vi "t값.vi"(5 "samples":i32=500, 7 "Time(S)":dbl=0.5, 8 "error in (no error)":errorcluster, 9 "c":dbl=0.001, 10 "r":dbl=40.0, 11 "v":dbl=800.0) -> (0 "error out":errorcluster, 2 "XY Graph":cluster{"Ramp Pattern":dbl[], dbl[]}[](graph), 3 "Waveform Graph":waveform(dbl)[](graph))   [LabVIEW 2019]
uses:
  <vilib>/Analysis/1siggen.llb/Ramp Pattern by Samples.vi
  <vilib>/Analysis/NI_AALBase.lvlib
panel:
  out "size(s) 2":i32
  out "size(s)":i32
  out "x/y":dbl
  out "output waveform":waveform(dbl)
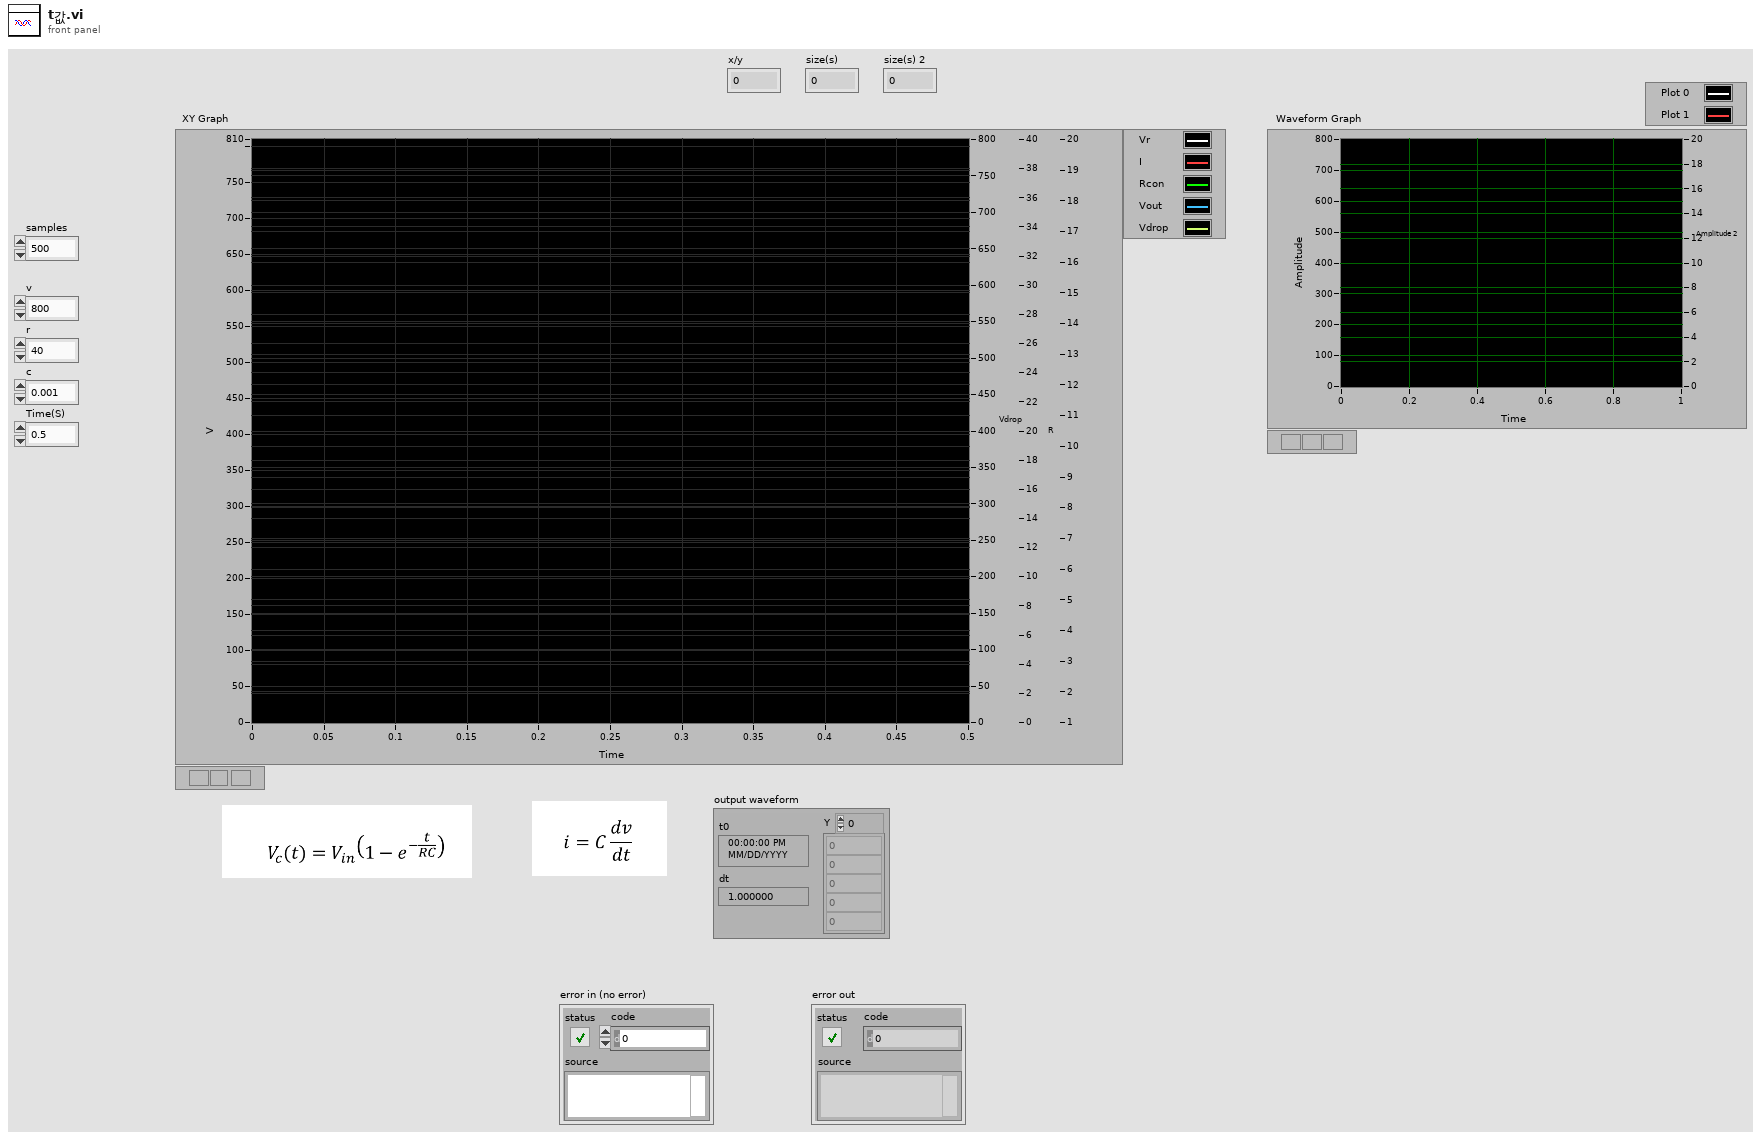
[diagram p1: front panel]
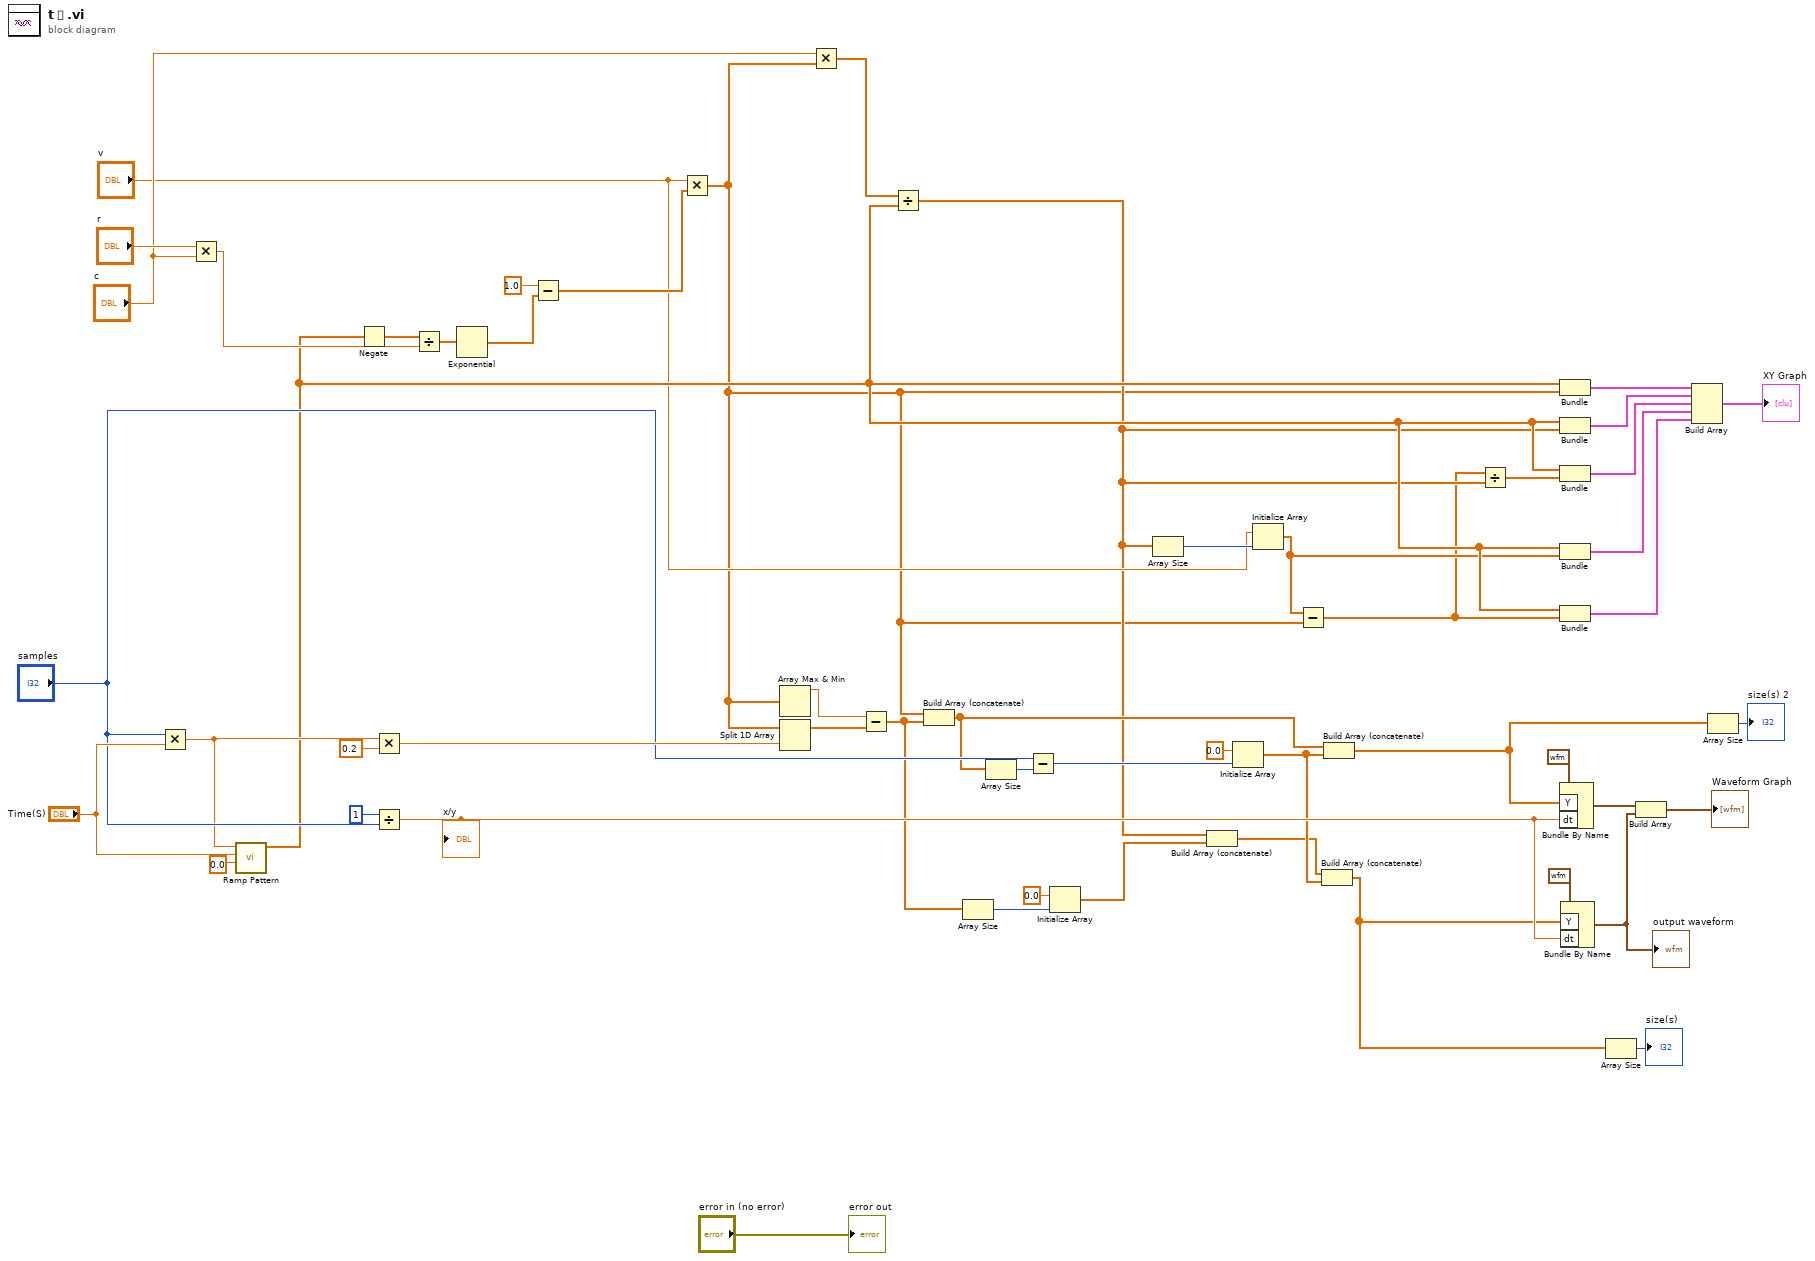
[diagram p0: block diagram]
diagram:
  n1 = Multiply(x="samples", y="Time(S)") -> (x*y=w34:dbl)
  n2 = Multiply(x="r", y="c") -> (x*y=w48:dbl)
  n3 = call-poly <vilib>:"Ramp Pattern.vi"("start"=0.0, "end"="Time(S)", "samples"=w34) -> ("Ramp Pattern"=w9:dbl[])  [unwired: 7 in, 1 out]
  n4 = Negate(x=w9) -> (-x=w51:dbl[])
  n5 = Multiply(x=w34, y=0.2) -> (x*y=w38:dbl)
  n6 = Divide(x=1, y="samples") -> (x/y=w40:dbl)
  "x/y" <- w40
  n7 = Divide(x=w51, y=w48) -> (x/y=w50:dbl[])
  n8 = Exponential(1:w50) -> (0:w7:dbl[])
  n9 = Subtract(x=1.0, y=w7) -> (x-y=w43:dbl[])
  n10 = Multiply(x="v", y=w43) -> (x*y=w2:dbl[])
  n11 = Array Max & Min(array=w2) -> (max value=w37:dbl)  [unwired: 3 out]
  n12 = Split 1D Array(array=w2, index=w38) -> (first subarray=w20:dbl[])  [unwired: 1 out]
  n13 = Multiply(x="c", y=w2) -> (x*y=w46:dbl[])
  n14 = Subtract(x=w37, y=w20) -> (x-y=w16:dbl[])
  n15 = Divide(x=w46, y=w9) -> (x/y=w4:dbl[])
  n16 = Build Array (concatenate)(w2, w16) -> (w18:dbl[])
  n17 = Array Size(array=w16) -> (size(s)=w19:i32)
  n18 = Array Size(array=w18) -> (size(s)=w35:i32)
  n19 = Subtract(x="samples", y=w35) -> (x-y=w27:i32)
  n20 = Initialize Array(0.0 ("element"), w19) -> (w15:dbl[])
  n21 = Array Size(array=w4) -> (size(s)=w10:i32)
  n22 = Build Array (concatenate)(w4, w15) -> (w14:dbl[])
  n23 = Initialize Array(0.0 ("element"), w27) -> (w17:dbl[])
  n24 = Initialize Array("v", w10) -> (w3:dbl[])
  n25 = Subtract(x=w3, y=w2) -> (x-y=w1:dbl[])
  n26 = Build Array (concatenate)(w14, w17) -> (w25:dbl[])
  n27 = Build Array (concatenate)(w18, w17) -> (w22:dbl[])
  n28 = Divide(x=w1, y=w4) -> (x/y=w6:dbl[])
  n29 = Bundle("Ramp Pattern"=w9, w2) -> (w45:cluster{"Ramp Pattern":dbl[], dbl[]})  [unwired: 1 in]
  n30 = Bundle("Ramp Pattern"=w9, w4) -> (w44:cluster{"Ramp Pattern":dbl[], dbl[]})  [unwired: 1 in]
  n31 = Bundle("Ramp Pattern"=w9, w6) -> (w13:cluster{"Ramp Pattern":dbl[], dbl[]})  [unwired: 1 in]
  n32 = Bundle("Ramp Pattern"=w9, w3) -> (w11:cluster{"Ramp Pattern":dbl[], dbl[]})  [unwired: 1 in]
  n33 = Bundle("Ramp Pattern"=w9, w1) -> (w8:cluster{"Ramp Pattern":dbl[], dbl[]})  [unwired: 1 in]
  n34 = Bundle By Name(cluster=waveform(dbl) {"t0"=timestamp(0 s since 1904-01-01), "dt"=0.0, "Y"=[]} ("data"), "Y"=w22, "dt"=w40) -> (w31:waveform(dbl))
  n35 = Bundle By Name(cluster=waveform(dbl) {"t0"=timestamp(0 s since 1904-01-01), "dt"=0.0, "Y"=[]} ("data"), "Y"=w25, "dt"=w40) -> (w29:waveform(dbl))
  "output waveform" <- w29
  n36 = Array Size(array=w25) -> (size(s)=→"size(s)":i32)
  n37 = Build Array(w31, w29) -> (→"Waveform Graph":waveform(dbl)[])
  n38 = Build Array(w45, w44, w13, w11, w8) -> (→"XY Graph":cluster{"Ramp Pattern":dbl[], dbl[]}[])
  n39 = Array Size(array=w22) -> (size(s)=→"size(s) 2":i32)
  "error out" <- "error in (no error)"
